vi "GLdrv_FILE_TRANS_OPEN.vi"(0 "Connection ID":T1, 11 "error in (no error)":errorcluster) -> (4 "Connection ID Out":T1, 6 "Error Code":i16, 15 "error out":errorcluster)   [LabVIEW 2017, in "GL860_Driver.lvlib"]
doc: "記録計本体内のファイルを転送します\nSOURceで設定したファイルをオープンします\n　：FILE:TRANS:OPEN? の後にレスポンスとして3バイトのステータス\nを返します\n1バイト目：　0x00：　予約バイト（使用しません）\n2バイト目：　16ビットステータスの上位8ビット\n3バイト目：　16ビットステータスの下位8ビット\n16ビットステータスの内容\nビット0：　1=エラーが発生／0=エラーは発生していない\nビット1～15ビット：　使用しません"
uses:
  GL860_Driver.lvlib
  ConnectionID.ctl
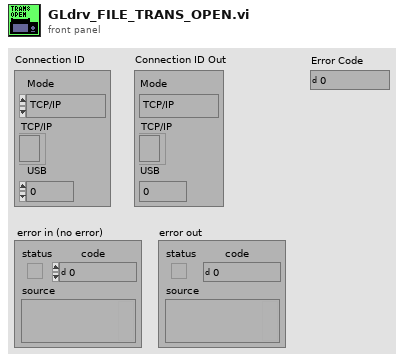
[diagram p1: front panel]
types:
  T1 = typedef "ConnectionID.ctl" = cluster{"Mode":enum16{"TCP/IP", "USB"}, "TCP/IP":refnum<k5>, "USB":i32}
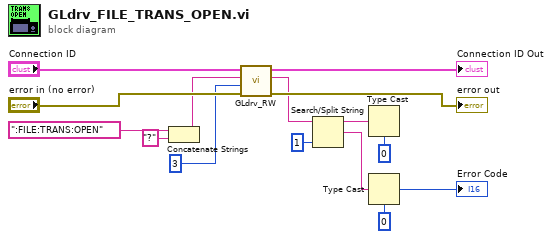
[diagram p0: block diagram]
diagram:
  n1 = Concatenate Strings(":FILE:TRANS:OPEN" ("Command"), "?" ("string")) -> (w9:string)
  n2 = call "GLdrv_RW.vi"("error in (no error)"="error in (no error)", "Count(0:[CR+LF])"=u32 3, "data in"=w9, "Connection ID"="Connection ID") -> ("error out"=→"error out":errorcluster, "data out"=w6:string, "Connection ID Out"=→"Connection ID Out":T1)  [unwired: 3 in, 2 out]
  n3 = Search/Split String(string=w6, offset (0)=1) -> (substring before match=w5:string, match + rest of string=w4:string)  [unwired: 2 out]
  n4 = Type Cast(type=u8 0 ("Status"), x=w5) -> ()  [unwired: 1 out]
  n5 = Type Cast(type=i16 0 ("Status"), x=w4) -> (*(type *) &x=→"Error Code":i16)
